vi "clear_all_relays.vi"   [LabVIEW 2011]
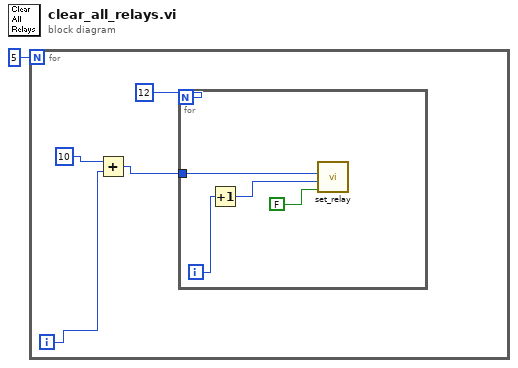
[diagram p0: block diagram]
diagram:
  n1 = for {
    N: 5 -> [_]
    i -> [w2]
    n2 = Add(x=10 ("y"), y=w2) -> (x+y=w4:i32)
    n3 = for {
      N: 12 -> [_]
      tunnel: w4 -> [w9]
      i -> [w6]
      n4 = Increment(x=w6) -> (x+1=w8:i32)
      n5 = call "set_relay.vi"("Slot"=w9, "Relay"=w8, "Relay Status"=FALSE) -> ()  [unwired: 3 out]
    }
  }
